vi "Oxygen Alarm.vi"() -> ()   [LabVIEW 2012]
uses:
  <vilib>/FieldPoint/Polymorphic Write.llb/FP Write (Float Array -IO).vi
  Instance          19 60Saved   Sensor Dynamic Data Logger + LN2 Control Backup copy .vi
  Instance           6 60Saved   Sensor Dynamic Data Logger + LN2 Control Backup copy .vi
  Instance          18 60Saved   Sensor Dynamic Data Logger + LN2 Control Backup copy .vi
  Instance           5 60Saved   Sensor Dynamic Data Logger + LN2 Control Backup copy .vi
  Instance           3 60Saved   Sensor Dynamic Data Logger + LN2 Control Backup copy .vi
  Instance           2 60Saved   Sensor Dynamic Data Logger + LN2 Control Backup copy .vi
  Instance          12 60Saved   Sensor Dynamic Data Logger + LN2 Control Backup copy .vi
  Instance           1 60Saved   Sensor Dynamic Data Logger + LN2 Control Backup copy .vi
  Instance          21 60Saved   Sensor Dynamic Data Logger + LN2 Control Backup copy .vi
  Instance          11 60Saved   Sensor Dynamic Data Logger + LN2 Control Backup copy .vi
  Instance          22 60Saved   Sensor Dynamic Data Logger + LN2 Control Backup copy .vi
  Instance           9 60Saved   Sensor Dynamic Data Logger + LN2 Control Backup copy .vi
  Instance           8 60Saved   Sensor Dynamic Data Logger + LN2 Control Backup copy .vi
  Instance          15 60Saved   Sensor Dynamic Data Logger + LN2 Control Backup copy .vi
  Instance          10 60Saved   Sensor Dynamic Data Logger + LN2 Control Backup copy .vi
  Instance           7 60Saved   Sensor Dynamic Data Logger + LN2 Control Backup copy .vi
  Instance           4 60Saved   Sensor Dynamic Data Logger + LN2 Control Backup copy .vi
  Instance          17 60Saved   Sensor Dynamic Data Logger + LN2 Control Backup copy .vi
  Instance          14 60Saved   Sensor Dynamic Data Logger + LN2 Control Backup copy .vi
  Instance          16 60Saved   Sensor Dynamic Data Logger + LN2 Control Backup copy .vi
  Instance          13 60Saved   Sensor Dynamic Data Logger + LN2 Control Backup copy .vi
panel:
  in  "124 upper mask":bool[](array[boolean])=[TRUE, TRUE, TRUE, TRUE, TRUE, TRUE, TRUE]
  in  "294 mask":bool[](array[boolean])=[TRUE, TRUE, TRUE, TRUE, TRUE, TRUE, TRUE]
  in  "124 lower mask":bool[](array[boolean])=[TRUE, TRUE, TRUE, TRUE, TRUE, TRUE, TRUE]
  out "Master Alarm 294":bool caption="Master Alarm  124"
  out "Master Alarm 124":bool caption="Master Alarm  124"
  out "Bldg 124 upper alarms":bool[](array[boolean]) caption="Red < 19.5% O2 2"
  in  "Reset Contros 124":bool
  out "Bldg 124 lower alarms":bool[](array[boolean]) caption="Red < 19.5% O2"
  in  "Reset Control 294":bool
  out "Bldg 294 alarms":bool[](array[boolean]) caption="RED < 19.5% O2"
  out "Bldg 294 Blkhd Valve Open":bool
  out "Bldg 294 Blkhd Valve Shut":bool
  out "Main Dewar Valve Shut":bool
  out "Main Dewar Valve Open":bool
  out "Air Flow sw 2":bool
  out "Air Flow sw 1":bool
  out "O2 Levels 124 LL":dynamicdata(graph) caption="Waveform Chart"
  out "O2 Levels 124 UL":dynamicdata(graph) caption="Waveform Chart"
  in  "stop":bool
  out "O2 Levels 294":dynamicdata(graph) caption="Waveform Chart"
  # "60T Pit"
  # "100T Pit"
  # "294 Above Pits"
  # "124UL Fill Station"
  # "Staff Lab"
  # "Cell 1"
  # "Cell 2"
  # "Cell 3"
  # "Cell 4"
  # "PPMS Lab"
  # "124LL Fill Station"
  # "100T Lab"
  # "Cell 5"
  # "20T Lab"
  # "Laser Lab"
  # "Cell 6"
  # "Cave"
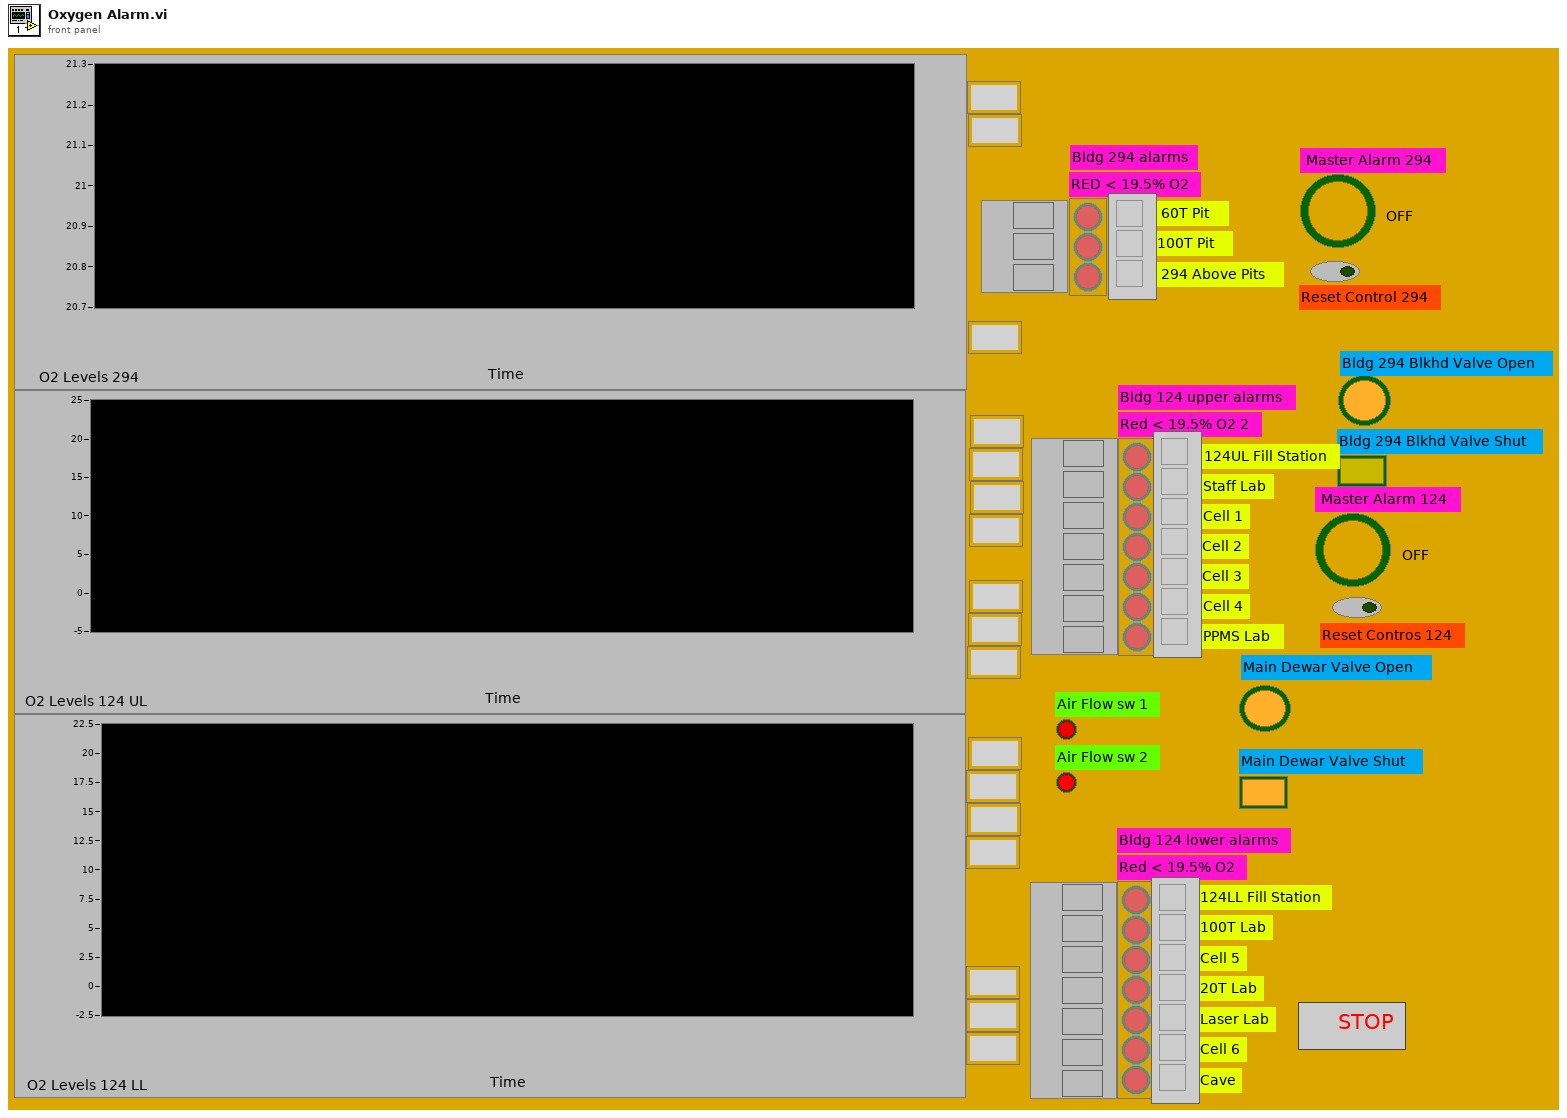
[diagram p1: front panel]
types:
  T1 = enum8{"Enabled", "Disabled", "Disabled and Grayed Out"}
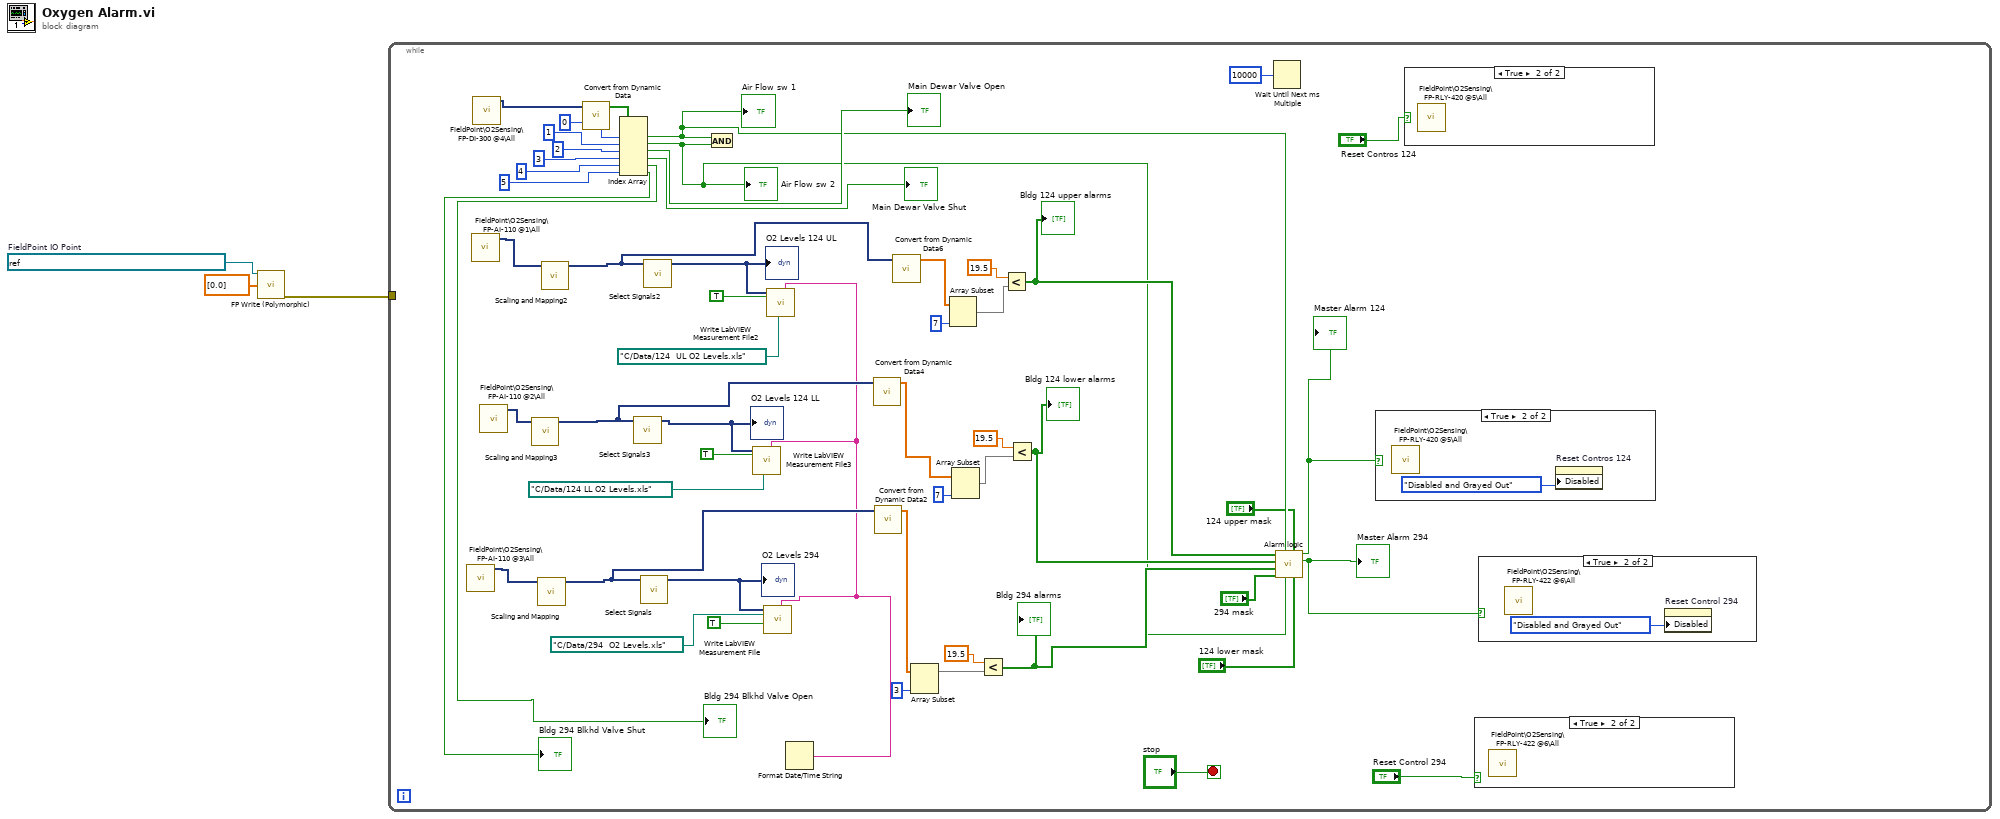
[diagram p0: block diagram]
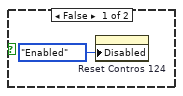
[diagram p3: hidden frame]
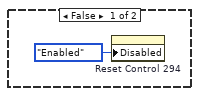
[diagram p5: hidden frame]
diagram:
  w3 = refnum<k21> "FieldPoint\\O2Sensing\\FP-2015 @0\\LED B"  # FieldPoint IO Point
  n1 = call-poly <vilib>:"FP Write (Polymorphic).vi"("FieldPoint IO Point In"=w3, "values"=dbl[] [0.0]) -> ("error out"=w1:errorcluster)  [unwired: 11 in, 2 out]
  n2 = while {
    tunnel: w1 -> [_]
    stop <- "stop" stop-if-true
    n3 = call "FieldPoint\\O2Sensing\\FP-AI-110 @3\\All"() -> ("Value out"=w24:dynamicdata)  [unwired: 4 in, 3 out]
    n4 = call "FieldPoint\\O2Sensing\\FP-AI-110 @1\\All"() -> ("Value out"=w25:dynamicdata)  [unwired: 4 in, 3 out]
    n5 = call "FieldPoint\\O2Sensing\\FP-DI-300 @4\\All"() -> ("Value out"=w23:dynamicdata)  [unwired: 4 in, 3 out]
    n6 = call "FieldPoint\\O2Sensing\\FP-AI-110 @2\\All"() -> ("Value out"=w22:dynamicdata)  [unwired: 4 in, 3 out]
    n7 = call "Scaling and Mapping3"("Signals"=w22) -> ("Scaled Signals"=w30:dynamicdata)  [unwired: 9 in, 1 out]
    n8 = call "Scaling and Mapping"("Signals"=w24) -> ("Scaled Signals"=w34:dynamicdata)  [unwired: 9 in, 1 out]
    n9 = call "Scaling and Mapping2"("Signals"=w25) -> ("Scaled Signals"=w27:dynamicdata)  [unwired: 9 in, 1 out]
    n10 = call "Convert from Dynamic Data"("Dynamic Data Type"=w23) -> ("Array"=w45:bool[])  [unwired: 3 in]
    n11 = Index Array(array=w45, index #1=0 ("index"), index #2=1 ("index"), index #3=2 ("index"), index #4=3 ("index"), index #5=4 ("index"), index #6=5 ("index")) -> (element #1=w8:bool, element #2=w7:bool, element #3=→"Main Dewar Valve Open":bool, element #4=→"Main Dewar Valve Shut":bool, element #5=→"Bldg 294 Blkhd Valve Open":bool, element #6=→"Bldg 294 Blkhd Valve Shut":bool)
    "Air Flow sw 1" <- w8
    "Air Flow sw 2" <- w7
    n12 = call "Select Signals3"("Signals"=w30) -> ("Signal Out"=w49:dynamicdata)  [unwired: 9 in, 1 out]
    "O2 Levels 124 LL" <- w49
    n13 = call "Select Signals"("Signals"=w34) -> ("Signal Out"=w55:dynamicdata)  [unwired: 9 in, 1 out]
    "O2 Levels 294" <- w55
    n14 = call "Select Signals2"("Signals"=w27) -> ("Signal Out"=w52:dynamicdata)  [unwired: 9 in, 1 out]
    "O2 Levels 124 UL" <- w52
    n15 = And(x=w8, y=w7) -> ()  [unwired: 1 out]
    n16 = Format Date/Time String() -> (date/time string=w26:string)  [unwired: 3 in]
    n17 = call "Write LabVIEW Measurement File3"("Comment"=w26, "File Name"=path "C:/Data/124 LL O2 Levels.xls", "Enable"=TRUE, "Signals"=w49) -> ()  [unwired: 5 in, 3 out]
    n18 = call "Write LabVIEW Measurement File"("Comment"=w26, "File Name"=path "C:/Data/294  O2 Levels.xls", "Enable"=TRUE, "Signals"=w55) -> ()  [unwired: 5 in, 3 out]
    n19 = call "Write LabVIEW Measurement File2"("Comment"=w26, "File Name"=path "C:/Data/124  UL O2 Levels.xls", "Enable"=TRUE, "Signals"=w52) -> ()  [unwired: 5 in, 3 out]
    n20 = call "Convert from Dynamic Data4"("Dynamic Data Type"=w30) -> ("Array"=w14:dbl[])  [unwired: 3 in]
    n21 = call "Convert from Dynamic Data2"("Dynamic Data Type"=w34) -> ("Array"=w33:dbl[])  [unwired: 3 in]
    n22 = call "Convert from Dynamic Data6"("Dynamic Data Type"=w27) -> ("Array"=w10:dbl[])  [unwired: 3 in]
    n23 = Array Subset(array=w33, length=3) -> (w18:dbl[])  [unwired: 1 in]
    n24 = Array Subset(array=w10, length=7) -> (w11:dbl[])  [unwired: 1 in]
    n25 = Array Subset(array=w14, length=7) -> (w13:dbl[])  [unwired: 1 in]
    n26 = Less?(x=19.5, y=w18) -> (x < y?=w21:bool[])
    "Bldg 294 alarms" <- w21
    n27 = Less?(x=19.5, y=w11) -> (x < y?=w19:bool[])
    "Bldg 124 upper alarms" <- w19
    n28 = Less?(x=19.5, y=w13) -> (x < y?=w20:bool[])
    "Bldg 124 lower alarms" <- w20
    n29 = Wait Until Next ms Multiple(millisecond multiple=u32 10000) -> ()  [unwired: 1 out]
    n30 = call "Alarm logic.vi"("124 lower mask"="124 lower mask", "124 upper mask"="124 upper mask", "Air Flow sw 2"=w7, "Air Flow sw 1"=w8, "294 mask"="294 mask", "Bldg 294 alarms"=w21, "Bldg 124 lower alarms"=w20, "Bldg 124 upper alarms"=w19) -> ("Master Alarm 294"=w9:bool, "Master Alarm  124"=w16:bool)  [unwired: 2 in]
    "Master Alarm 124" <- w16
    "Master Alarm 294" <- w9
    n31 = case shown="True" w16 {
      frame False {
        n32 = property on="Reset Contros 124" class="Bool"("Disabled"=T1."Enabled") -> ()  [unwired: 2 in, 2 out]
      }
      frame True {
        n33 = call "FieldPoint\\O2Sensing\\FP-RLY-420 @5\\All"() -> ()  [unwired: 6 in, 2 out]
        n34 = property on="Reset Contros 124" class="Bool"("Disabled"=T1."Disabled and Grayed Out") -> ()  [unwired: 2 in, 2 out]
      }
    }
    n35 = case shown="True" "Reset Contros 124" {
      frame False {
      }
      frame True {
        n36 = call "FieldPoint\\O2Sensing\\FP-RLY-420 @5\\All"() -> ()  [unwired: 6 in, 2 out]
      }
    }
    n37 = case shown="True" "Reset Control 294" {
      frame False {
      }
      frame True {
        n38 = call "FieldPoint\\O2Sensing\\FP-RLY-422 @6\\All"() -> ()  [unwired: 6 in, 2 out]
      }
    }
    n39 = case shown="True" w9 {
      frame False {
        n40 = property on="Reset Control 294" class="Bool"("Disabled"=T1."Enabled") -> ()  [unwired: 2 in, 2 out]
      }
      frame True {
        n41 = call "FieldPoint\\O2Sensing\\FP-RLY-422 @6\\All"() -> ()  [unwired: 6 in, 2 out]
        n42 = property on="Reset Control 294" class="Bool"("Disabled"=T1."Disabled and Grayed Out") -> ()  [unwired: 2 in, 2 out]
      }
    }
  }
